vi "Get ProtoFile Messages.vi"(8 "error in (no error)":errorcluster, 11 "Protofile ref in":u64) -> (0 "error out":errorcluster, 2 "ProtoFile Messages":u64[](array[numeric]), 3 "Protofile ref out":u64)   [LabVIEW 2019, in "gRPC Template Creation Utility.lvlib"]
uses:
  gRPC Template Creation Utility.lvlib
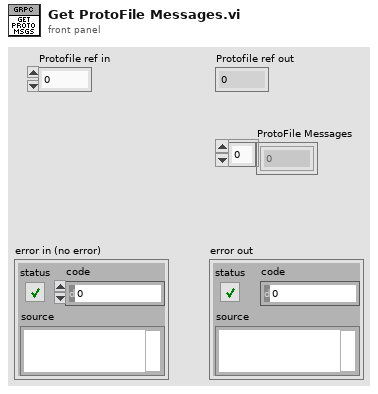
[diagram p1: front panel]
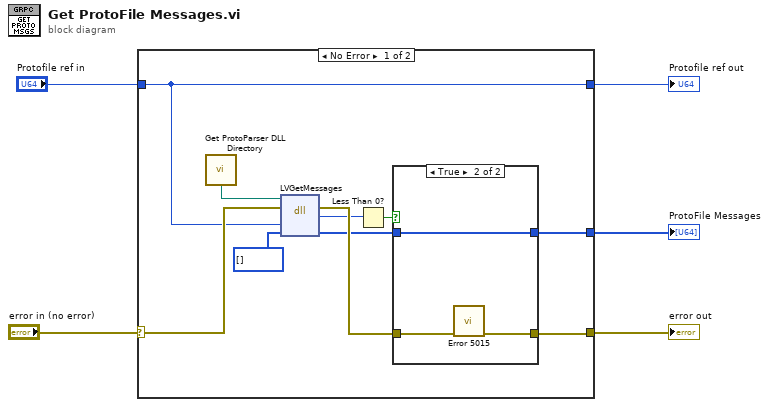
[diagram p0: block diagram]
diagram:
  n1 = case shown="No Error" "error in (no error)" {
    selector: "error in (no error)" -> [w13 w21]
    tunnel: "Protofile ref in" -> [w12 w22]
    tunnel: [w12 w22] -> w3
    tunnel: [w11 w21] -> w2
    tunnel: [w6 _] -> w1
    frame No Error {
      n2 = call "Get ProtoParser DLL Directory.vi"() -> ("Proto Parser Directory"=w14:path)
      n3 = dll-call lib="C:/Users/XEnderMD/Desktop/LV gRPC/labview source/gRPC Scripting Tools/Proto Parser API/dll/labview_grpc_generator.dll" fn="LVGetMessages"(path in=w14, error in=w13, "protoDescription"=w12, "messages"=u64[] []) -> (error out=w10:errorcluster, "return type"=w9:i32, "messages"=w7:u64[])  [unwired: 2 in, 1 out]
      n4 = Less Than 0?(x=w9) -> (x < 0?=w8:bool)
      n5 = case shown="True" w8 {
        tunnel: [w16 w20] -> w11
        tunnel: w10 -> [w16 w19]
        tunnel: w7 -> [w17 w18]
        tunnel: [w17 w18] -> w6
        frame False {
        }
        frame True {
          n6 = call "Error 5015.vi"("error in (no error)"=w19) -> ("error out"=w20:errorcluster)  [unwired: 10 in]
        }
      }
    }
    frame Error {
    }
  }
  "ProtoFile Messages" <- w1
  "Protofile ref out" <- w3
  "error out" <- w2
